vi "Com_Matrix220_Reading Trigger.vi"(8 "error in":errorcluster, 11 "Buffer Data In":T1) -> (0 "error out":errorcluster, 3 "Buffer Data Out":T1)   [LabVIEW 2016]
uses:
  Data Def/Com_Matrix220_Buffer Data.ctl
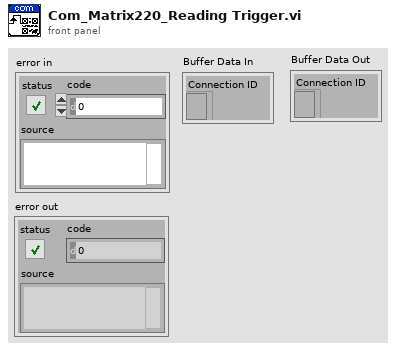
[diagram p1: front panel]
types:
  T1 = typedef "Com_Matrix220_Buffer Data.ctl" = cluster{"Connection ID":refnum<k5>}
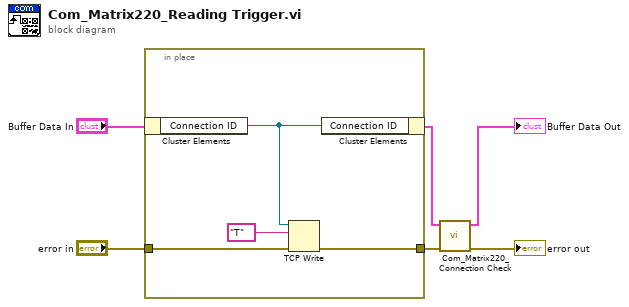
[diagram p0: block diagram]
diagram:
  n1 = in-place {
    in-place-border: "error in" -> [w8]
    in-place-border: [w7] -> w3
    n2 = in-place-cluster #1("Buffer Data In") -> ("Connection ID"=w10:refnum<k5>)
    n3 = TCP Write(connection ID=w10, data in="T", error in (no error)=w8) -> (error out=w7:errorcluster)  [unwired: 1 in, 2 out]
    n4 = in-place-cluster #1("Connection ID"=w10) -> (w4:T1)
  }
  n5 = call "Com_Matrix220_Connection Check.vi"("error in"=w3, "Buffer Data In"=w4) -> ("error out"=→"error out":errorcluster, "Buffer Data Out"=→"Buffer Data Out":T1)  [unwired: 7 in, 1 out]
